vi "WhileLoop Get Selector C Call.vi"(8 "error in":errorcluster, 11 "reference":refnum<vi>) -> (0 "error out":errorcluster, 3 "WhileLoop Selector C string":string)   [LabVIEW 2014]
doc: "Generates WhileLoop condition based on wire connected to end terminal. It takes it's name and generte statement:\ndo{\n}while([WhileLoop Selector]);"
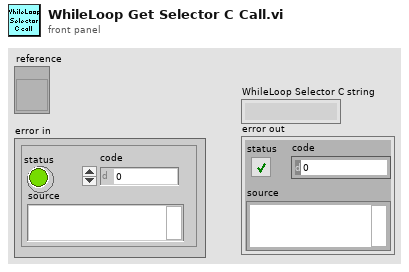
[diagram p1: front panel]
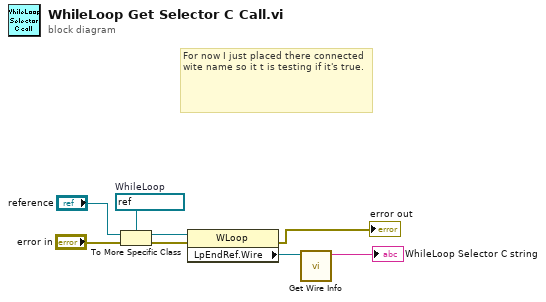
[diagram p0: block diagram]
diagram:
  w8 = refnum<vi> refnum  # WhileLoop
  # "For now I just placed there connected wite name so it t is testing if it's true."
  n1 = To More Specific Class(target class=w8, reference="reference", error in="error in") -> (specific class reference=w6:refnum<vi>, error out=w5:errorcluster)
  n2 = property class="WLoop"(reference=w6, error in=w5) -> (error out=→"error out":errorcluster, "LpEndRef.Wire"=w3:refnum<vi>)  [unwired: 1 out]
  n3 = call "Get Wire Info.vi"("Wire"=w3) -> ("wire label"=→"WhileLoop Selector C string":string)  [unwired: 9 in, 1 out]
